vi "Shallow Copy Priv.vi"(0 "Tree Dictionary In":variant, 5 "Unique ID":string, 11 "error in":errorcluster) -> (4 "Tree Dictionary Out":variant, 8 "ID":string, 15 "error out":errorcluster)   [LabVIEW 2016, in "Tree Manager.lvclass"]
uses:
  Tree Manager.lvclass
  Typedefs/Tree.ctl
  Tree Data/Tree Data.lvclass
  <vilib>/Utility/error.llb/Error Cluster From Error Code.vi
  <vilib>/ErrorRing/Error Ring.xnode
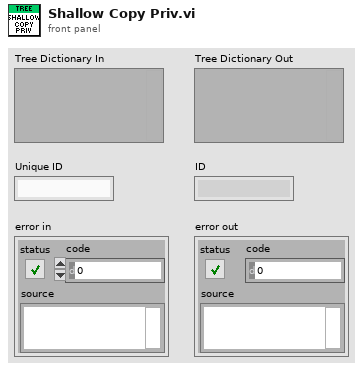
[diagram p1: front panel]
types:
  T1 = typedef "Tree Manager.lvclass/Tree.ctl" = cluster{"Unique ID":string, "Parent ID":string, "Child IDs":string[], "Data":variant, "Name":string}
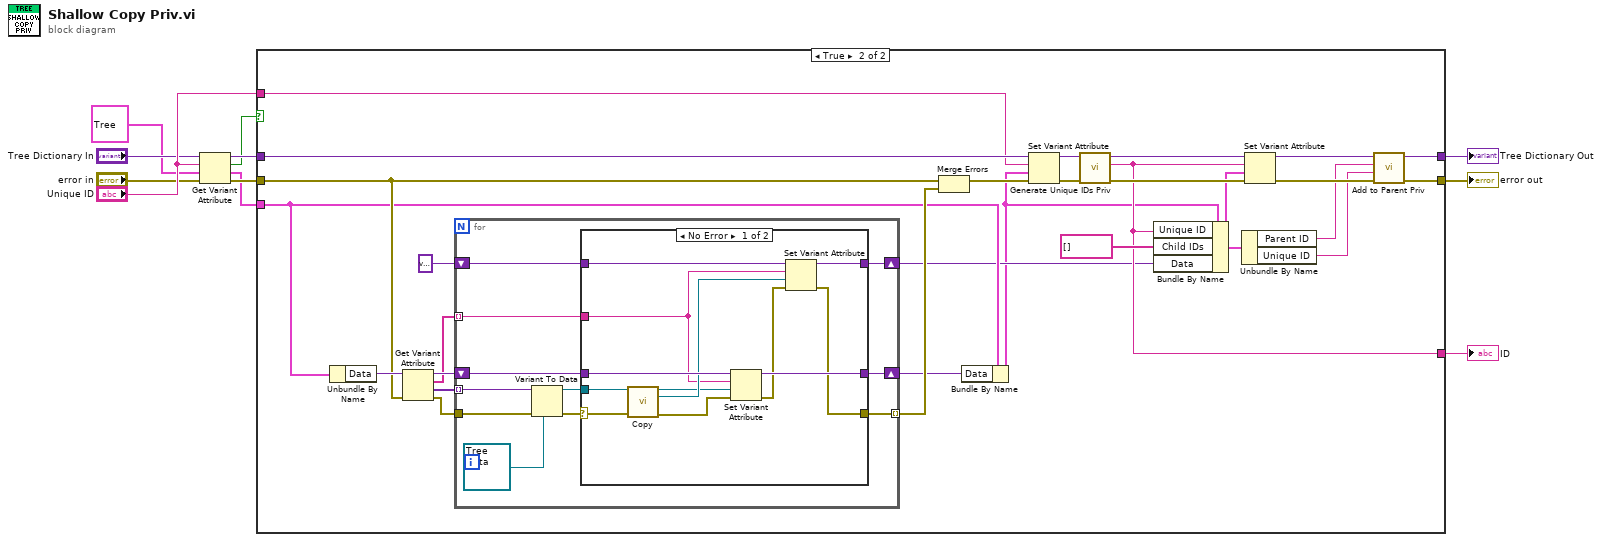
[diagram p0: block diagram]
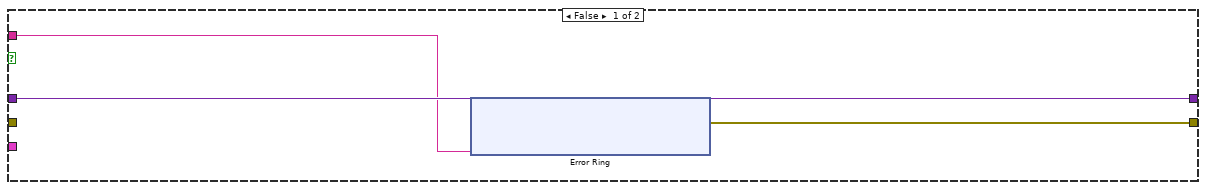
[diagram p2: hidden frame]
diagram:
  n1 = Get Variant Attribute(Variant="Tree Dictionary In", name="Unique ID", default value (empty Variant)=T1 {"Unique ID"="", "Parent ID"="", "Child IDs"=[], "Data"=variant, "Name"=""} ("Cluster of class private data"), error in="error in") -> (duplicate Variant=w5:variant, found=w3:bool, value=w4:T1, error out=w6:errorcluster)
  n2 = case shown="True" w3 {
    tunnel: w4 -> [_ w35]
    tunnel: w5 -> [w14 w37]
    tunnel: w6 -> [_ w39]
    tunnel: [w12 w26] -> w9
    tunnel: [w14 w25] -> w8
    tunnel: "Unique ID" -> [w13 w29]
    tunnel: [_ w46] -> w2
    frame False {
      n3 = xnode "Error Ring"("parameter 0"=w13) -> ("error out"=w12:errorcluster)
    }
    frame True {
      n4 = Unbundle By Name(w35) -> ("Data"=w45:variant)
      n5 = Get Variant Attribute(Variant=w45, error in=w39) -> (duplicate Variant=w43:variant, names=w40:string[], values=w44:variant[], error out=w42:errorcluster)  [unwired: 2 in]
      n6 = for {
        tunnel: w44 -> [w60] mode=indexing
        shift-right: [w52] -> w34
        shift-left: w43 -> [w55]
        shift-right: [w53] -> w33
        shift-left: variant ("duplicate variant") -> [w54]
        tunnel: w40 -> [w51] mode=indexing
        tunnel: w42 -> [w56]
        tunnel: [w50] -> w38 mode=indexing
        n7 = Variant To Data(error in=w56, type=refnum<class "Tree Data.lvclass"> refnum ("Tree Data.lvclass"), Variant=w60) -> (data=w57:refnum<class "Tree Data.lvclass">, error out=w58:errorcluster)
        n8 = case shown="No Error" w58 {
          selector: w58 -> [w64 _]
          tunnel: w57 -> [w72 _]
          tunnel: w55 -> [w71 w73]
          tunnel: w54 -> [w70 w74]
          tunnel: [w69 w74] -> w53
          tunnel: [w68 w73] -> w52
          tunnel: w51 -> [w65 _]
          tunnel: [w61 _] -> w50
          frame No Error {
            n9 = call-dynamic "Copy.vi"("Tree Data"=w72, "Error In"=w64) -> ("Original"=w66:refnum<class "Tree Data.lvclass">, "Copy"=w67:refnum<class "Tree Data.lvclass">, "Error Out"=w63:errorcluster)  [unwired: 11 in]
            n10 = Set Variant Attribute(Variant=w71, name=w65, value=w66, error in=w63) -> (Variant out=w68:variant, error out=w62:errorcluster)  [unwired: 1 out]
            n11 = Set Variant Attribute(Variant=w70, name=w65, value=w67, error in=w62) -> (Variant out=w69:variant, error out=w61:errorcluster)  [unwired: 1 out]
          }
          frame Error {
          }
        }
      }
      n12 = Merge Errors(w39, w38) -> (w36:errorcluster)
      n13 = Bundle By Name(cluster=w35, "Data"=w34) -> (w30:T1)
      n14 = Set Variant Attribute(Variant=w37, name=w29, value=w30, error in=w36) -> (Variant out=w32:variant, error out=w31:errorcluster)  [unwired: 1 out]
      n15 = call "Generate Unique IDs Priv.vi"("Error In"=w31, "Tree Dictionary"=w32) -> ("Error Out"=w47:errorcluster, "First ID"=w46:string, "Tree Dictionary Out"=w49:variant)  [unwired: 6 in, 1 out]
      n16 = Bundle By Name(cluster=w30, "Unique ID"=w46, "Child IDs"=string[] [], "Data"=w33) -> (w24:T1)
      n17 = Unbundle By Name(w24) -> ("Parent ID"=w23:string, "Unique ID"=w22:string)
      n18 = Set Variant Attribute(Variant=w49, name=w46, value=w24, error in=w47) -> (Variant out=w28:variant, error out=w27:errorcluster)  [unwired: 1 out]
      n19 = call "Add to Parent Priv.vi"("Error In"=w27, "Unique ID"=w22, "Parent ID"=w23, "Tree Dictionary"=w28) -> ("Error Out"=w26:errorcluster, "Tree Dictionary Out"=w25:variant)  [unwired: 6 in]
    }
  }
  "error out" <- w9
  "Tree Dictionary Out" <- w8
  "ID" <- w2
